vi "Remove.vi"(8 "error in (no error)":errorcluster, 10 "Key":string, 11 "Dictionary in":refnum<class "Dictionary.lvclass">) -> (0 "error out":errorcluster, 1 "Success?":bool, 3 "Dictionary out":refnum<class "Dictionary.lvclass">)   [LabVIEW 2018, in "Application.lvlib" / "Dictionary.lvclass"]
uses:
  Dictionary.lvclass
  Dictionary.lvclass/Dictionary.ctl
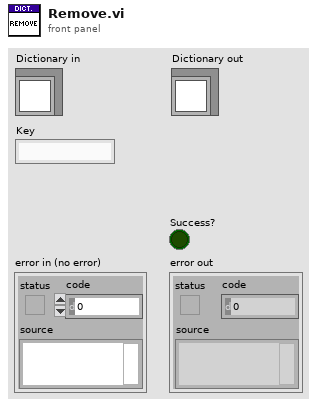
[diagram p1: front panel]
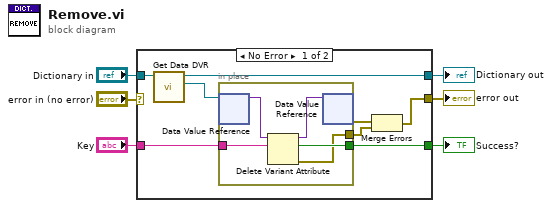
[diagram p0: block diagram]
diagram:
  n1 = case shown="No Error" "error in (no error)" {
    selector: "error in (no error)" -> [_ w21]
    tunnel: [w7 w21] -> w5
    tunnel: [w12 w20] -> w3
    tunnel: "Dictionary in" -> [w14 w20]
    tunnel: "Key" -> [w11 _]
    tunnel: [w10 _] -> w1
    frame No Error {
      n2 = call "Get Data DVR.vi"("Dictionary in"=w14) -> ("Data DVR"=w13:refnum<data-value>, "Dictionary out"=w12:refnum<class "Dictionary.lvclass">)  [unwired: 8 in, 1 out]
      n3 = in-place {
        in-place-border: w11 -> [w18]
        in-place-border: [w17] -> w10
        in-place-border: [w16] -> w8
        n4 = in-place-dvr #1(w13) -> (w19:variant)  [unwired: 1 out]
        n5 = Delete Variant Attribute(6:w18, 7:w19) -> (0:w16:errorcluster, 2:w17:bool, 3:w15:variant)  [unwired: 1 in]
        n6 = in-place-dvr #1(w15) -> (w9:errorcluster)  [unwired: 1 out]
      }
      n7 = Merge Errors(w9, w8) -> (w7:errorcluster)
    }
    frame Error {
    }
  }
  "error out" <- w5
  "Dictionary out" <- w3
  "Success?" <- w1
